vi "Read Unlock Publication Msg.vi"(11 "IModel in":refnum<class "IModel.lvclass">) -> (2 "Pre-Addressed Unlock Msg":refnum<class "Unlock Publication Msg.lvclass">)   [LabVIEW 2020, in "MVA Framework.lvlib" / "IModel.lvlib" / "IModel.lvclass"]
doc: "读取解锁发布消息"
uses:
  IModel.lvclass
  IMediator/IMediator Messages/Unlock Publication Msg/Unlock Publication Msg.lvclass
  IModel.lvclass/IModel.ctl
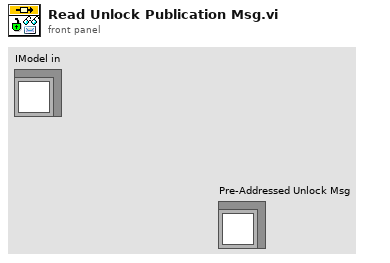
[diagram p1: front panel]
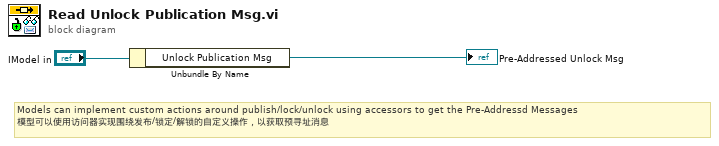
[diagram p0: block diagram]
diagram:
  # "Models can implement custom actions around publish/lock/unlock using accessors to get the Pre-Addressd Messages\n模型可以使用访问器实现围绕发布/锁定/解锁的自定义操作，以获取预寻址消息"
  n1 = Unbundle By Name("IModel in") -> ("Unlock Publication Msg"=→"Pre-Addressed Unlock Msg":refnum<class "Unlock Publication Msg.lvclass">)
